vi "WM Output Random Seas (math only).vi"(2 "error in (no error)":errorcluster, 4 "Start up":bool, 6 "Run":bool, 7 "Task ID In":u32, 8 "End":bool, 9 "Sub Buffer Size":dbl format="%.2f", 10 "Sampling Rate":dbl format="%.2f", 11 "Input Time Series":dbl[](array[numeric]) format="%.2f") -> (0 "End Out":bool, 3 "Buffer":dbl[](array[numeric]) format="%.2f")   [LabVIEW 2012]
uses:
  <vilib>/Analysis/1siggen.llb/Ramp Pattern by Samples.vi
  <vilib>/Analysis/NI_AALBase.lvlib
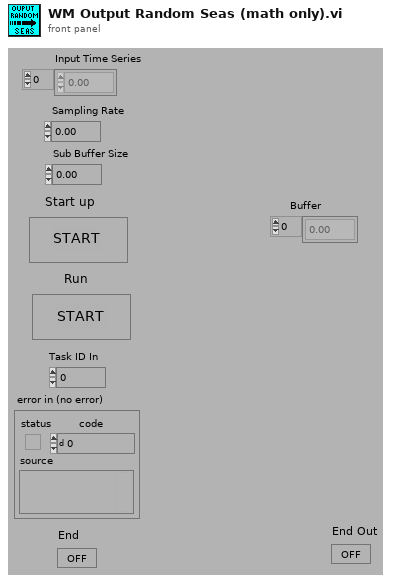
[diagram p1: front panel]
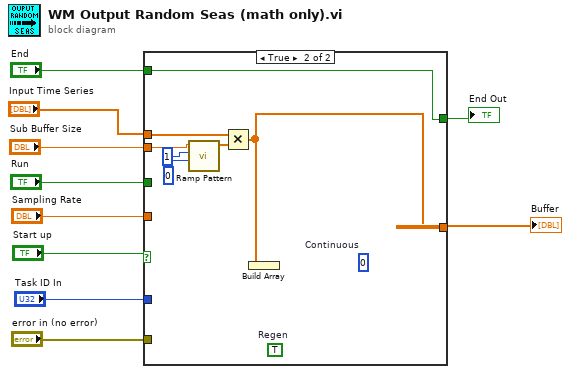
[diagram p0: block diagram]
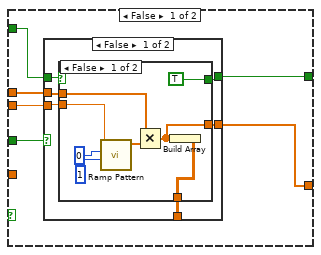
[diagram p2: hidden frame]
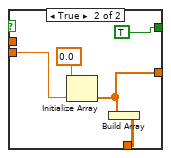
[diagram p3: hidden frame]
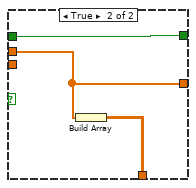
[diagram p4: hidden frame]
diagram:
  n1 = case shown="True" "Start up" {
    tunnel: "Input Time Series" -> [w16 w42]
    tunnel: "Sub Buffer Size" -> [w15 w43]
    tunnel: [w14 w40] -> w9
    tunnel: "Run" -> [w13 _]
    tunnel: "error in (no error)" -> [_ _]
    tunnel: "Task ID In" -> [_ _]
    tunnel: "Sampling Rate" -> [_ _]
    tunnel: "End" -> [w12 w39]
    tunnel: [w11 w39] -> w1
    frame False {
      n2 = case shown="False" w13 {
        tunnel: w16 -> [w22 w38]
        tunnel: w15 -> [w21 _]
        tunnel: [w20 w38] -> w14
        tunnel: [w19 w37] -> _
        tunnel: w12 -> [w18 w36]
        tunnel: [w17 w36] -> w11
        frame False {
          n3 = case shown="False" w18 {
            tunnel: w22 -> [w30 _]
            tunnel: w21 -> [w29 w33]
            tunnel: [w28 w35] -> w20
            tunnel: [w27 w34] -> w19
            tunnel: [TRUE TRUE] -> w17
            frame False {
              n4 = call-poly <vilib>:"Ramp Pattern.vi"("start"=i8 1, "end"=i8 0, "samples"=w29) -> ("Ramp Pattern"=w24:dbl[])  [unwired: 7 in, 1 out]
              n5 = Multiply(x=w30, y=w24) -> (x*y=w28:dbl[])
              n6 = Build Array(w28) -> (w27:dbl[][])
            }
            frame True {
              n7 = Initialize Array(0.0 ("Element Data"), w33) -> (w35:dbl[])
              n8 = Build Array(w35) -> (w34:dbl[][])
            }
          }
        }
        frame True {
          n9 = Build Array(w38) -> (w37:dbl[][])
        }
      }
    }
    frame True {
      (unwired) TRUE  # Regen
      (unwired) 0  # Continuous
      n10 = call-poly <vilib>:"Ramp Pattern.vi"("start"=i8 0, "end"=i8 1, "samples"=w43) -> ("Ramp Pattern"=w41:dbl[])  [unwired: 7 in, 1 out]
      n11 = Multiply(x=w42, y=w41) -> (x*y=w40:dbl[])
      n12 = Build Array(w40) -> ()  [unwired: 1 out]
    }
  }
  "Buffer" <- w9
  "End Out" <- w1
